vi "RM-connect-axis.vi"(8 "Error in":errorcluster caption="Error in (no error)", 9 "baud rate (bps)":u32=9600, 10 "axisNo":i32, 11 "VISA引用句柄输入":refnum<visa-resource-name>) -> (0 "Error out":errorcluster, 3 "MB_Master_Serial输出":refnum<class "MB_Master_Serial.lvclass">)   [LabVIEW 2014]
uses:
  <vilib>/Plasmionique/MB Master/MB_Master_Serial/MB_Master_Serial.lvclass
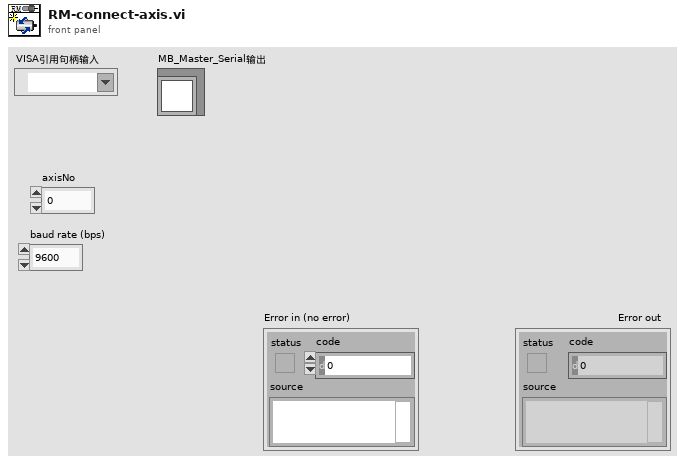
[diagram p1: front panel]
types:
  T1 = cluster{"baud rate (bps)":u32, "stop bits":u16, "parity":u16, "flow control":u16, "timeout":u32, "retries":i32}
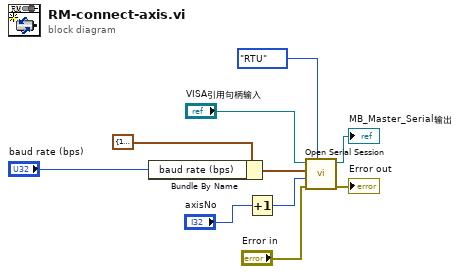
[diagram p0: block diagram]
diagram:
  n1 = Bundle By Name(cluster=T1 {"baud rate (bps)"=19200, "stop bits"=10, "parity"=0, "flow control"=0, "timeout"=1000, "retries"=1} ("Serial Config"), "baud rate (bps)"="baud rate (bps)") -> (w5:T1)
  n2 = Increment(x="axisNo") -> (x+1=w8:i32)
  n3 = call <vilib>:"Open Serial Session.vi"("Mode (RTU)"=enum16{"RTU", "ASCII"}."RTU", "Error in"="Error in", "Slave ID"=w8, "Serial Config"=w5, "VISA Resource"="VISA引用句柄输入") -> ("Error out"=→"Error out":errorcluster, "MB_Serial session"=→"MB_Master_Serial输出":refnum<class "MB_Master_Serial.lvclass">)  [unwired: 5 in]
